vi "ARCUS STAGE COMMAND.vi"(6 "READ BYTES":u32=1024, 8 "error in (no error)":errorcluster, 10 "COMMANDS":string[](array[string]), 11 "OBJECT IN":refnum<visa-resource-name>) -> (0 "error out":errorcluster, 2 "OUTPUT":string[](array[string]), 3 "OBJECT OUT":refnum<visa-resource-name>)   [LabVIEW 2018]
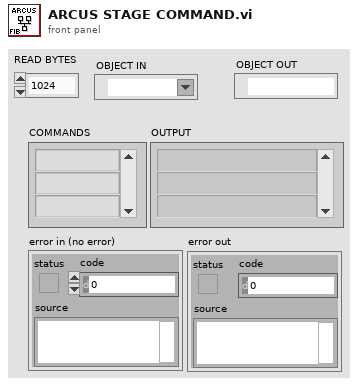
[diagram p1: front panel]
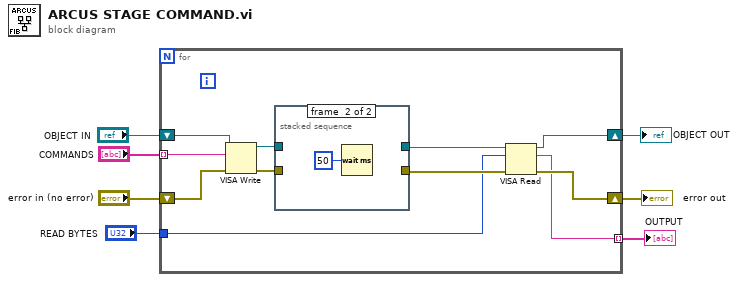
[diagram p0: block diagram]
diagram:
  n1 = for {
    tunnel: "COMMANDS" -> [w8] mode=indexing
    tunnel: "READ BYTES" -> [w11]
    shift-right: [w10] -> w2
    shift-left: "OBJECT IN" -> [w18]
    shift-right: [w16] -> w5
    shift-left: "error in (no error)" -> [w17]
    tunnel: [w9] -> w1 mode=indexing
    n2 = VISA Write(VISA resource name=w18, write buffer=w8, error in (no error)=w17) -> (VISA resource name out=w14:refnum<visa-resource-name>, error out=w12:errorcluster)  [unwired: 1 out]
    n3 = stacked-sequence {
      tunnel: [w20 _] -> w15
      tunnel: w14 -> [w20 _]
      tunnel: [w19 _] -> w13
      tunnel: w12 -> [w19 _]
      frame #0 {
      }
      frame #1 {
        n4 = Wait (ms)(milliseconds to wait=u32 50) -> ()  [unwired: 1 out]
      }
    }
    n5 = VISA Read(VISA resource name=w15, byte count=w11, error in (no error)=w13) -> (VISA resource name out=w10:refnum<visa-resource-name>, read buffer=w9:string, error out=w16:errorcluster)  [unwired: 1 out]
  }
  "OBJECT OUT" <- w2
  "error out" <- w5
  "OUTPUT" <- w1
